vi "似生長曲線 actan.vi"() -> ()   [LabVIEW 2015]
uses:
  <vilib>/Utility/file.llb/Write Delimited Spreadsheet (DBL).vi
  <vilib>/Utility/file.llb/Read Delimited Spreadsheet (DBL).vi
panel:
  out "read":errorcluster
  out "read":cluster{dbl[], dbl[]}(graph)
  out "write":errorcluster
  out "atan":cluster{dbl[], dbl[]}(graph)
  out "cos":cluster{dbl[], dbl[]}(graph)
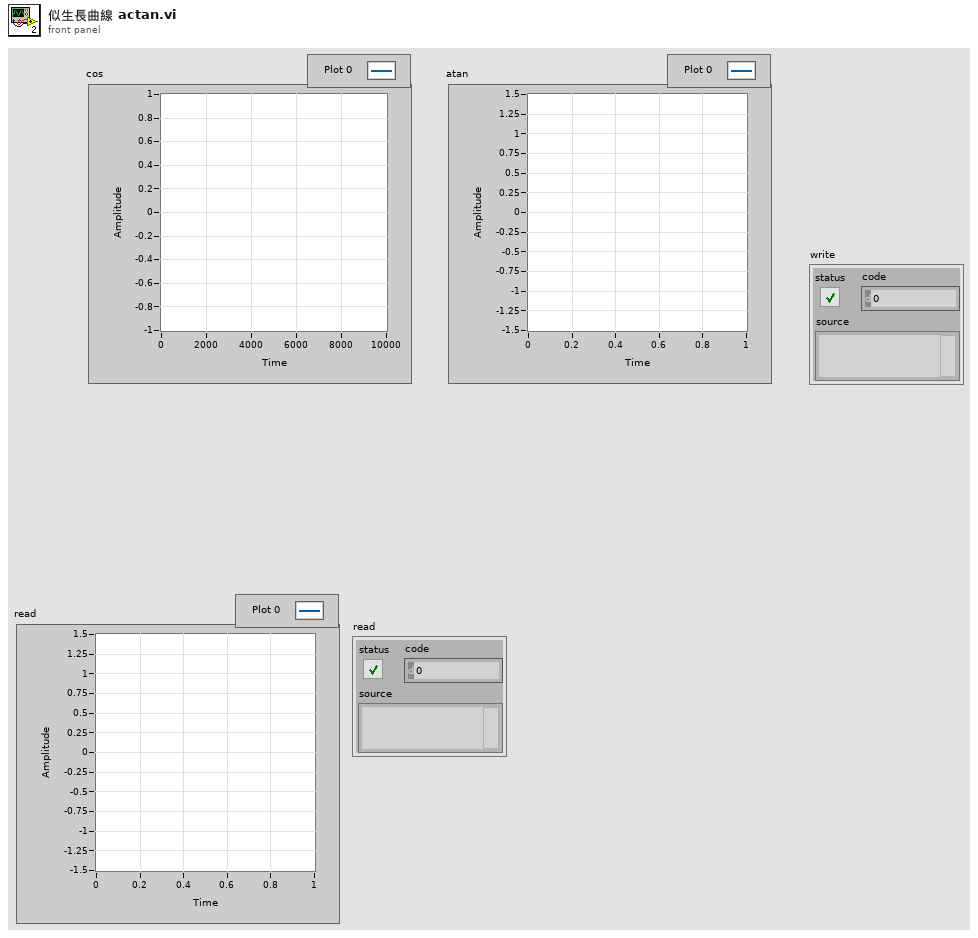
[diagram p1: front panel]
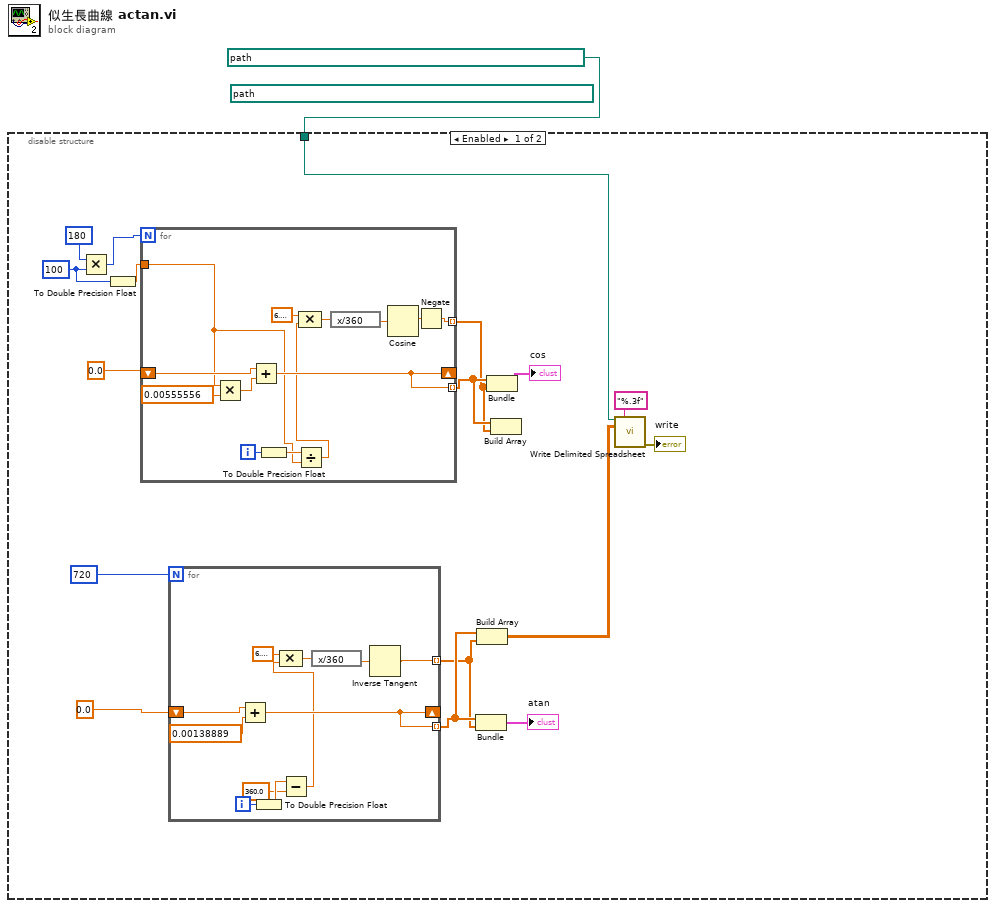
[diagram p0: block diagram]
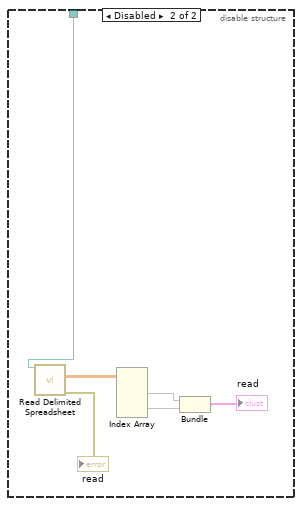
[diagram p2: hidden frame]
diagram:
  (unwired) path "C:/Users/user/Desktop/0.0labview 電腦程式專用/atan-arraytest"
  n1 = disable-structure shown="Enabled" {
    disable-tunnel: path "C:/Users/user/Desktop/0.0labview 電腦程式專用/cos-arraytest" -> [w9 w48]
    frame Enabled {
      w3 = 100 ("y")
      n2 = Multiply(x=180, y=w3) -> (x*y=w2:i32)
      n3 = To Double Precision Float(number=w3) -> (double precision float=w4:dbl)
      n4 = for {
        N: w2 -> [_]
        tunnel: [w24] -> w11 mode=indexing
        shift-right: [w27] -> _
        shift-left: 0.0 -> [w28]
        tunnel: [w27] -> w12 mode=indexing
        tunnel: w4 -> [w19]
        i -> [w31]
        n5 = Multiply(x=w19, y=0.00555556) -> (x*y=w23:dbl)
        n6 = Add(x=w28, y=w23) -> (x+y=w27:dbl)
        n7 = To Double Precision Float(number=w31) -> (double precision float=w20:dbl)
        n8 = Divide(x=w20, y=w19) -> (x/y=w21:dbl)
        n9 = Compound Arithmetic op=MULTIPLY(6.283185307179586, w21) -> (w29:dbl)
        n10 = expression code="x/360"(w29) -> (w26:dbl)
        n11 = Cosine(x=w26) -> (cos(x)=w25:dbl)
        n12 = Negate(x=w25) -> (-x=w24:dbl)
      }
      n13 = for {
        N: 720 -> [_]
        tunnel: [w38] -> w7 mode=indexing
        shift-right: [w35] -> _
        shift-left: 0.0 -> [w37]
        tunnel: [w35] -> w8 mode=indexing
        i -> [w42]
        n14 = Add(x=w37, y=0.00138889) -> (x+y=w35:dbl)
        n15 = To Double Precision Float(number=w42) -> (double precision float=w34:dbl)
        n16 = Subtract(x=w34, y=360.0) -> (x-y=w32:dbl)
        n17 = Compound Arithmetic op=MULTIPLY(6.283185307179586, w32) -> (w40:dbl)
        n18 = expression code="x/360"(w40) -> (w39:dbl)
        n19 = Inverse Tangent(1:w39) -> (0:w38:dbl)
      }
      n20 = Bundle(w8, w7) -> (→"atan":cluster{dbl[], dbl[]})  [unwired: 1 in]
      n21 = Build Array(w8, w7) -> (w6:dbl[][])
      n22 = Bundle(w12, w11) -> (→"cos":cluster{dbl[], dbl[]})  [unwired: 1 in]
      n23 = Build Array(w12, w11) -> ()  [unwired: 1 out]
      n24 = call-poly <vilib>:"Write Delimited Spreadsheet.vi"("file path (dialog if empty)"=w9, "format (%.3f)"="%.3f", "2D data"=w6) -> ("error out"=→"write":errorcluster)  [unwired: 11 in, 1 out]
    }
    frame Disabled {
      n25 = call-poly <vilib>:"Read Delimited Spreadsheet.vi"("file path (dialog if empty)"=w48) -> ("all rows"=w47:dbl[][], "error out"=→"read":errorcluster)  [unwired: 9 in, 4 out]
      n26 = Index Array(array=w47) -> (element #1=w46:dbl[], element #2=w45:dbl[])  [unwired: 4 in]
      n27 = Bundle("all rows"=w46, "all rows"=w45) -> (→"read":cluster{"all rows":dbl[], "all rows":dbl[]})  [unwired: 1 in]
    }
  }
